vi "MtrPwrMapping.vi"(10 "OldPwr":dbl, 11 "NewMaxPwr":dbl) -> (3 "NewPwr":dbl)   [LabVIEW 2017]
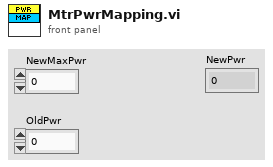
[diagram p1: front panel]
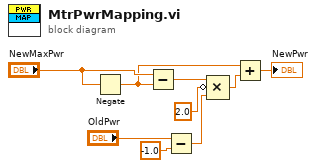
[diagram p0: block diagram]
diagram:
  n1 = Negate(x="NewMaxPwr") -> (-x=w8:dbl)
  n2 = Subtract(x="NewMaxPwr", y=w8) -> (x-y=w3:dbl)
  n3 = Subtract(x="OldPwr", y=-1.0) -> (x-y=w2:dbl)
  n4 = Compound Arithmetic op=MULTIPLY(w3, invert 2.0, w2) -> (w4:dbl)
  n5 = Add(x=w8, y=w4) -> (x+y=→"NewPwr":dbl)
